vi "Reset.vi"(8 "error in (no error)":errorcluster, 11 "Timed Out in":refnum<class "Timed Out.lvclass">) -> (0 "error out":errorcluster, 3 "State Actor out":refnum<class "State Actor.lvclass">)   [LabVIEW 2024, in "Sample State Actor.lvlib" / "Timed Out.lvclass"]
uses:
  Timed Out.lvclass
  State Actor/State Actor.lvclass
  Idle/Idle.lvclass
  C:/Users/ottoa/OneDrive/Desktop/working copies/stateActor/src/State Actor/State Actor.lvclass
  Timed Out.lvclass/Timed Out.ctl
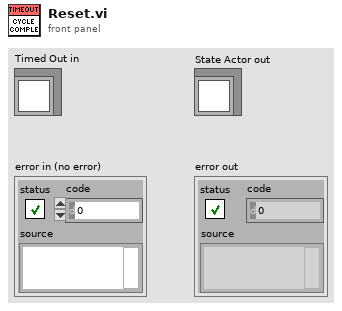
[diagram p1: front panel]
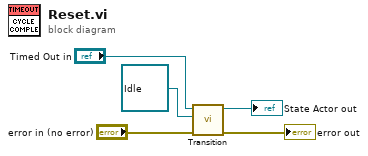
[diagram p0: block diagram]
diagram:
  n1 = call-dynamic "Transition.vi"("error in (no error)"="error in (no error)", "Target State Actor in"=refnum<class "Idle.lvclass"> refnum ("Sample State Actor.lvlib:Idle.lvclass"), "State Actor in"="Timed Out in") -> ("error out"=→"error out":errorcluster, "State Actor out"=→"State Actor out":refnum<class "State Actor.lvclass">)  [unwired: 7 in]
